vi "Update NV.vi"(8 "error in (no error)":errorcluster, 11 "Stand in":refnum<class "Stand.lvclass">) -> (0 "error out":errorcluster)   [LabVIEW 2019, in "Stand.lvclass"]
uses:
  Stand.lvclass
  <vilib>/NI/Modbus Library/API/Master/Modbus Master.lvclass
  Stand.lvclass/Stand.ctl
  <vilib>/NI/Modbus Library/API/Wrapper/Create TCP Master.vi
  NeedleValve_class/NeedleValve.lvclass
  <vilib>/NI/Modbus Library/API/Wrapper/API Main.lvlib
panel:
  out "stop":bool
  in  "cont stop":u32
  in  "reset":bool
  in  "max dont change":i32=200
  out "Waveform Chart 3":i32(graph)
  out "Waveform Chart 2":i32(graph)
  out "Waveform Chart":u32(graph)
  out "count":u32
  out "change direction":bool
  out "dt":u32
  out "error out 2":errorcluster
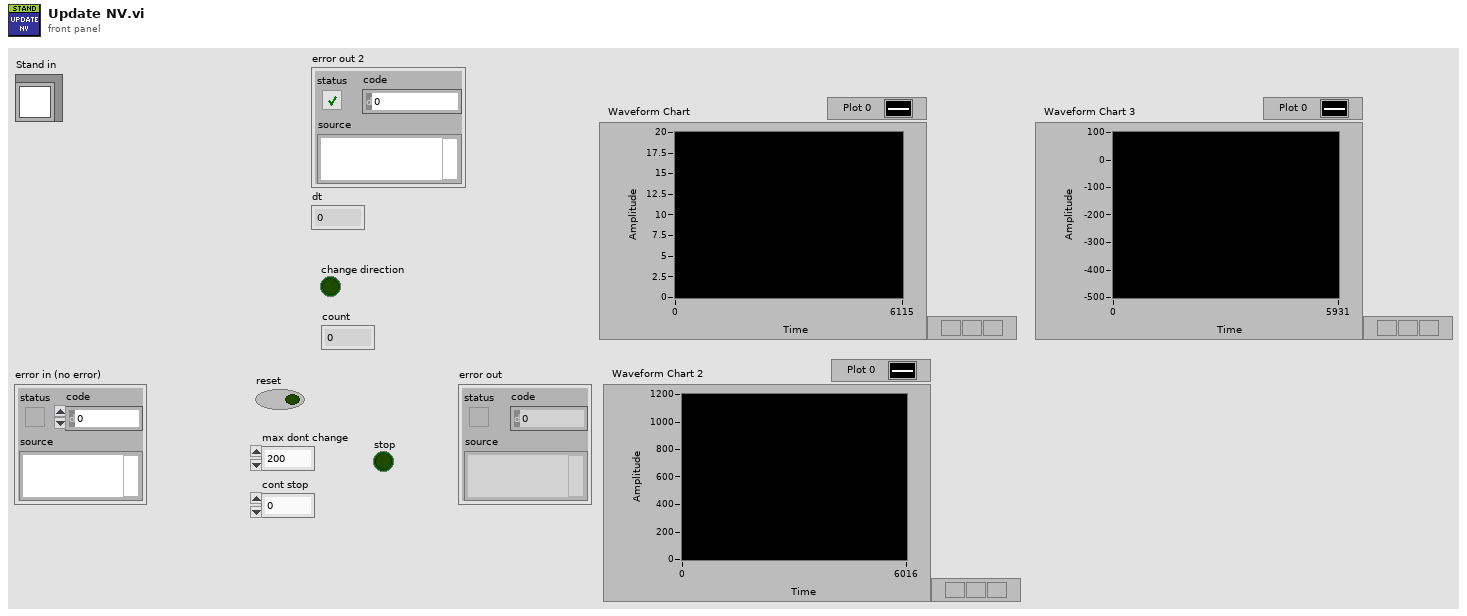
[diagram p1: front panel]
types:
  T1 = typedef "Needle Valve Data.ctl" = cluster{"Engine State":T2, "StateValveModbus":T3, "Alarms":T4, "RAW":i32, "Angele":dbl, "Step":i32, "Encoder":i32, "Kinematic":T5, "Limits":T6, "EncoderMax":i32, "Counter Max Dont Update":i32, "EncoderMin":i32, "Counter Min Dont Update":i32, "Prepere Counter":i32, "STEP INIT":i32, "offset - Angel":dbl}
  T2 = typedef "MB_ENGINE.lvclass/Engine State.ctl" = u16
  T3 = typedef "Needle Valve State.ctl" = enum16{"STOPED", "CLOSED", "OPENED", "OPENING", "CLOSING", "FULL_CLOSE", "PREP_OPEN"}
  T4 = typedef "MB_ENGINE.lvclass/Engine Alarms.ctl" = cluster{"OL":bool, "TF":bool, "STL":bool, "OCP":bool, "CPUV":bool, "UVLO":bool, "SPI_ERROR":bool, "Fault":bool, "OL 2":bool, "TF 2":bool, "STL 2":bool, "OCP 2":bool, "CPUV 2":bool, "UVLO 2":bool, "reserved":bool, "InitDone":bool}
  T5 = typedef "MB_ENGINE.lvclass/Settings.ctl" = cluster{"ACC Steps Per Sec^2":u16, "DEC Steps Per Sec^2":u16, "Min Velosity Step Per Sec":u16, "Max Velosity Step Per Sec":u16, "MicroStep":u16}
  T6 = typedef "MB_ENGINE.lvclass/Limits Status.ctl" = cluster{"Fault 2 Switch":bool, "Fault 1 Switch":bool, "Center(Home)":bool, "Lower Limit":bool, "Upper Limit":bool}
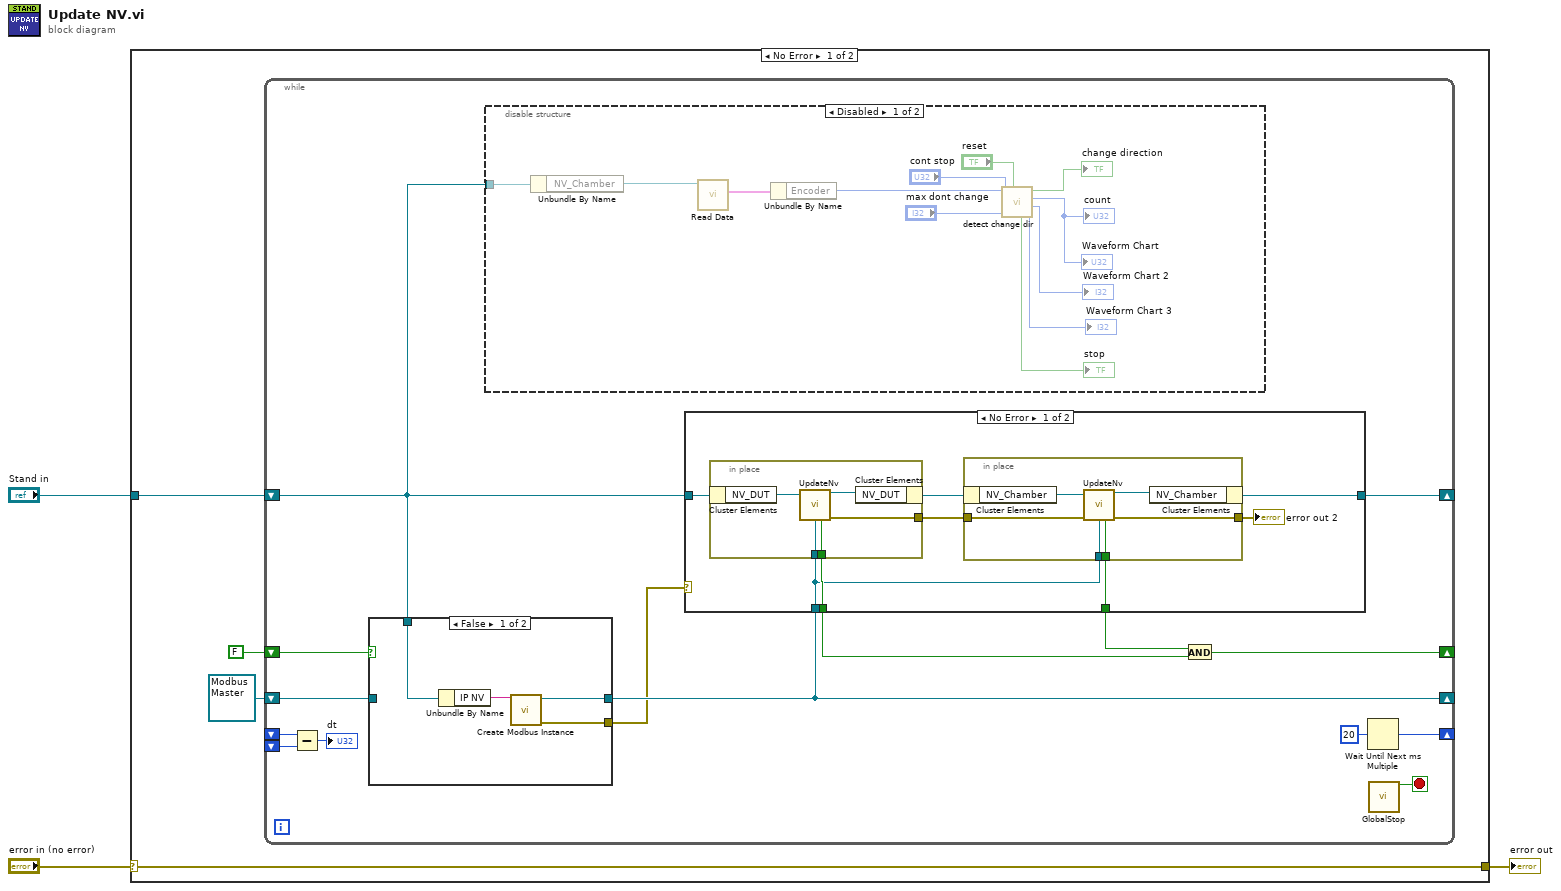
[diagram p0: block diagram]
diagram:
  n1 = case shown="No Error" "error in (no error)" {
    selector: "error in (no error)" -> [w7 w60]
    tunnel: [w7 w60] -> w2
    tunnel: "Stand in" -> [w6 _]
    frame No Error {
      n2 = while {
        shift-right: [w19] -> _
        shift-left: refnum<class "Modbus Master.lvclass"> refnum ("TCP master instance") -> [w16]
        shift-right: [w18] -> _
        shift-left: FALSE -> [w17]
        shift-right: [w15] -> _
        shift-left: w6 -> [w8]
        shift-right: [w12] -> _
        shift-left: _ -> [w11]
        shift-left: _ -> [w10]
        stop <- w22 stop-if-true
        n3 = Subtract(x=w11, y=w10) -> (x-y=→"dt":u32)
        n4 = case shown="False" w17 {
          tunnel: w8 -> [w58 _]
          tunnel: [w56 w59] -> w19
          tunnel: w16 -> [_ w59]
          tunnel: [w55 _] -> w14
          frame False {
            n5 = Unbundle By Name(w58) -> ("IP NV"=w57:string)
            n6 = call-poly <vilib>:"Create Modbus Instance.vi"("address"=w57) -> ("error out"=w55:errorcluster, "TCP master instance"=w56:refnum<class "Modbus Master.lvclass">)  [unwired: 9 in]
          }
          frame True {
          }
        }
        n7 = disable-structure shown="Disabled" {
          disable-tunnel: w8 -> [w34 _]
          frame Disabled {
            n8 = Unbundle By Name(w34) -> ("NV_Chamber"=w33:refnum<class "NeedleValve.lvclass">)
            n9 = call "Read Data.vi"("NeedleValve in"=w33) -> ("data value"=w32:T1)  [unwired: 10 in]
            n10 = Unbundle By Name(w32) -> ("Encoder"=w31:i32)
            n11 = call "detect change dir.vi"("reset"="reset", "cont stop"="cont stop", "max dont change"="max dont change", "in"=w31) -> ("x-y"=→"Waveform Chart 3":i32, "dont change count"=→"Waveform Chart 2":i32, "count"=→"count" →"Waveform Chart":u32, "change direction"=→"change direction":bool, "stop"=→"stop":bool)  [unwired: 3 in]
          }
          frame Enabled {
          }
        }
        n12 = case shown="No Error" w14 {
          tunnel: w8 -> [w40 w54]
          tunnel: [w39 _] -> w21
          tunnel: [w38 _] -> w20
          tunnel: w19 -> [w37 _]
          tunnel: [w36 w54] -> w15
          frame No Error {
            n13 = in-place {
              in-place-border: [w51] -> w41
              in-place-border: w37 -> [w50]
              in-place-border: [w49] -> w39
              n14 = in-place-cluster #1(w40) -> ("NV_DUT"=w53:refnum<class "NeedleValve.lvclass">)
              n15 = call "UpdateNv.vi"("Pump_1AI_1DO_2DI in"=w53, "modbus"=w50) -> ("Pump_1AI_1DO_2DI out"=w52:refnum<class "NeedleValve.lvclass">, "Connected"=w49:bool, "error out"=w51:errorcluster)  [unwired: 11 in]
              n16 = in-place-cluster #1("NV_DUT"=w52) -> (w42:refnum<class "Stand.lvclass">)
            }
            n17 = in-place {
              in-place-border: w41 -> [w46]
              in-place-border: w37 -> [w45]
              in-place-border: [w44] -> w35
              in-place-border: [w43] -> w38
              n18 = in-place-cluster #2(w42) -> ("NV_Chamber"=w48:refnum<class "NeedleValve.lvclass">)
              n19 = call "UpdateNv.vi"("Pump_1AI_1DO_2DI in"=w48, "error in (no error)"=w46, "modbus"=w45) -> ("Pump_1AI_1DO_2DI out"=w47:refnum<class "NeedleValve.lvclass">, "Connected"=w43:bool, "error out"=w44:errorcluster)  [unwired: 10 in]
              n20 = in-place-cluster #2("NV_Chamber"=w47) -> (w36:refnum<class "Stand.lvclass">)
            }
            "error out 2" <- w35
          }
          frame Error {
          }
        }
        n21 = And(x=w20, y=w21) -> (x .and. y?=w18:bool)
        n22 = Wait Until Next ms Multiple(millisecond multiple=u32 20) -> (millisecond timer value=w12:u32)
        n23 = call "GlobalStop.vi"() -> ("Stop"=w22:bool)  [unwired: 15 in]
      }
    }
    frame Error {
    }
  }
  "error out" <- w2
